vi "Create Command.vi"(10 "Cue Information":T1 {"Channels"."Intensity" min=0.0 max=100.0 step=1.0 format="%#.0f"}) -> (3 "Record out":refnum<class "Record.lvclass">)   [LabVIEW 2010, in "Record.lvclass"]
doc: "This instance of Create Command.vi writes the value of the Cue Information input to the data stored within Record.lvclass."
uses:
  Record.lvclass
  Controls/tlc_Cue_Information.ctl
  Controls/channel.ctl
  Record.lvclass/Record.ctl
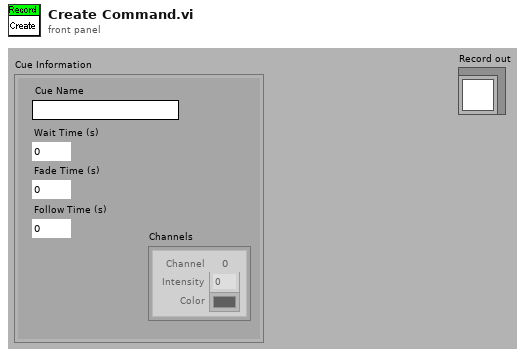
[diagram p1: front panel]
types:
  T1 = typedef "tlc_Cue_Information.ctl" = cluster{"Cue Name":string, "Wait Time (s)":u32, "Fade Time (s)":u32, "Follow Time (s)":u32, "Channels":T2[][]}
  T2 = typedef "channel.ctl" = cluster{"Intensity":dbl, " Color":u32, "Channel":i32}
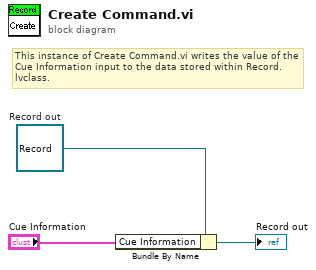
[diagram p0: block diagram]
diagram:
  w3 = refnum<class "Record.lvclass"> refnum  # Record out
  # "This instance of Create Command.vi writes the value of the Cue Information input to the data stored within Record.lvclass."
  n1 = Bundle By Name "Bundle By Name"(cluster=w3, "Cue Information"="Cue Information") -> (→"Record out":refnum<class "Record.lvclass">)
